vi "NI9205_Global.vi"() -> ()   [LabVIEW 2016]
panel:
  out "NI9205 Signals":dynamicdata(graph)
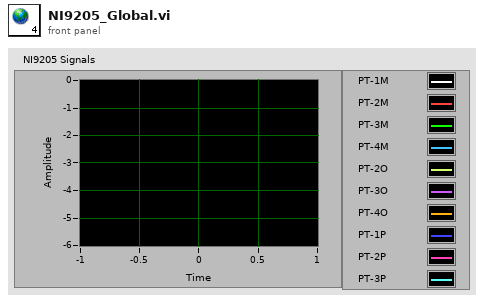
[diagram p1: front panel]
diagram:
